vi "FTW-JSON-ObjectManip-AddPair-Boolean.vi"(0 "Input JSON Object":string, 5 "Key":string, 7 "Value":bool, 11 "error in":errorcluster) -> (4 "Output JSON Object":string, 15 "error out":errorcluster)   [LabVIEW 2013]
uses:
  FTW-JSON.lvclass
panel:
  # "Inputs"
  # "Outputs"
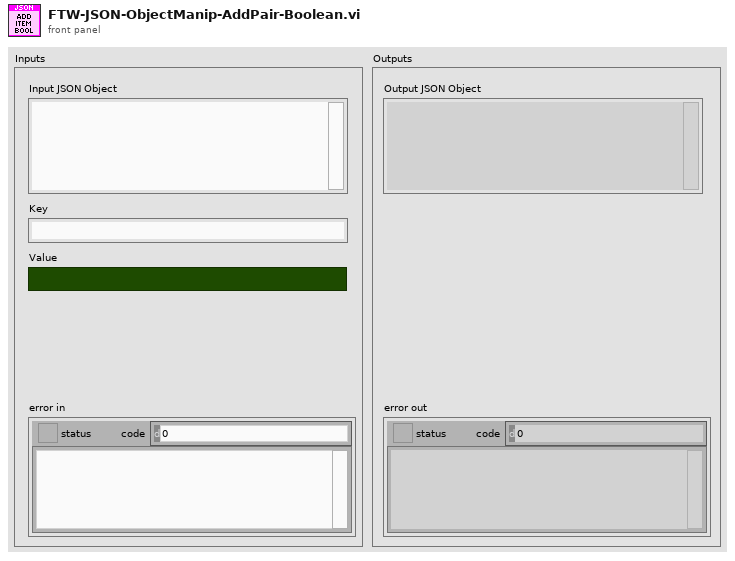
[diagram p1: front panel]
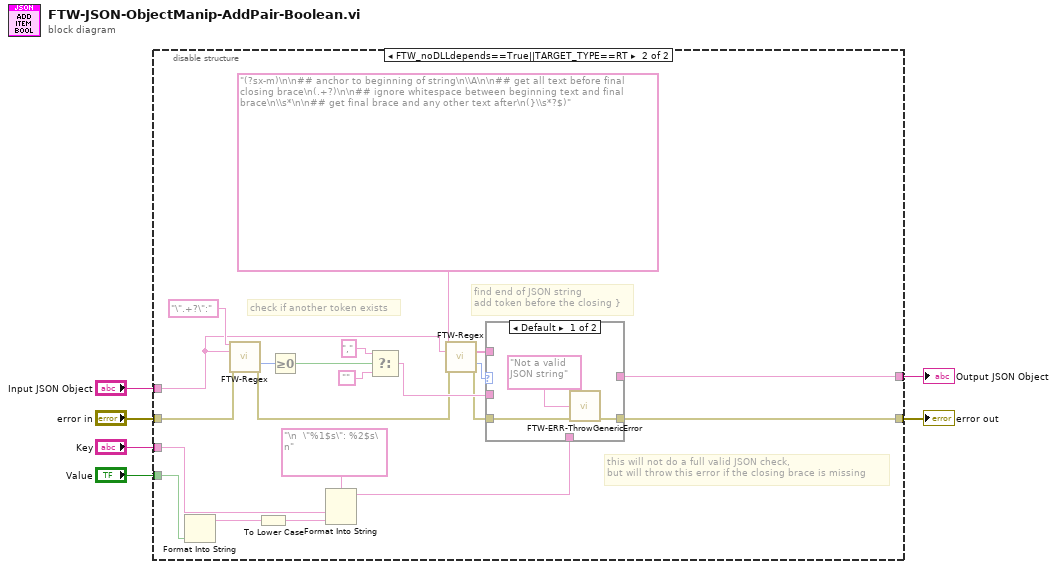
[diagram p0: block diagram]
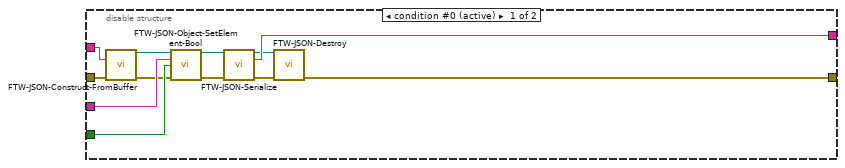
[diagram p2: hidden frame]
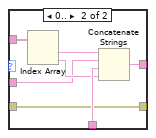
[diagram p3: hidden frame]
diagram:
  n1 = disable-structure shown="FTW_noDLLdepends==True||TARGET_TYPE==RT" {
    disable-tunnel: "Key" -> [w18 w31]
    disable-tunnel: "Value" -> [w17 w21]
    disable-tunnel: "Input JSON Object" -> [w16 w23]
    disable-tunnel: "error in" -> [w15 w30]
    disable-tunnel: [w14 w32] -> w2
    disable-tunnel: [w13 w33] -> w1
    frame condition #0 (active) {
      n2 = call "FTW-JSON-Construct-FromBuffer.vi"("JSON String (UTF-8)"=w16, "error in"=w15) -> ("JSON Object"=w10:refnum<class "FTW-JSON.lvclass">, "error out"=w8:errorcluster)  [unwired: 12 in]
      n3 = call "FTW-JSON-Object-SetElement-Bool.vi"("JSON Object"=w10, "Key"=w18, "Value"=w17, "error in"=w8) -> ("JSON Object out"=w9:refnum<class "FTW-JSON.lvclass">, "error out"=w7:errorcluster)  [unwired: 10 in]
      n4 = call "FTW-JSON-Serialize.vi"("JSON Object"=w9, "error in"=w7) -> ("JSON Object out"=w12:refnum<class "FTW-JSON.lvclass">, "JSON String (UTF-8)"=w13:string, "error out"=w11:errorcluster)  [unwired: 11 in]
      n5 = call "FTW-JSON-Destroy.vi"("JSON Object"=w12, "error in"=w11) -> ("error out"=w14:errorcluster)  [unwired: 13 in]
    }
    frame condition #1 {
      # "this will not do a full valid JSON check,\nbut will throw this error if the closing brace is missing"
      # "find end of JSON string\nadd token before the closing }"
      # "check if another token exists"
      n6 = Format Into String(w21) -> (resulting string=w20:string)  [unwired: 3 in, 1 out]
      n7 = call "FTW-Regex.vi"("Regular Expression"="\".+?\":" ("format string"), "Input String"=w23, "error in"=w30) -> ("Offset after Match"=w22:i32, "error out"=w28:errorcluster)  [unwired: 8 in, 3 out]
      n8 = To Lower Case(string=w20) -> (all lower case string=w19:string)
      n9 = Greater Or Equal To 0?(x=w22) -> (x >= 0?=w35:bool)
      n10 = Format Into String(format string="\n  \"%1$s\": %2$s\n", w31, w19) -> (resulting string=w38:string)  [unwired: 2 in, 1 out]
      n11 = Select(t="," ("format string"), s=w35, f="") -> (s? t:f=w39:string)
      n12 = call "FTW-Regex.vi"("Regular Expression"="(?sx-m)\n\n## anchor to beginning of string\n\\A\n\n## get all text before final closing brace\n(.+?)\n\n## ignore whitespace between beginning text and final brace\n\\s*\n\n## get final brace and any other text after\n(}\\s*?$)" ("format string"), "Input String"=w23, "error in"=w28) -> ("Submatches"=w25:string[], "Offset after Match"=w24:i32, "error out"=w27:errorcluster)  [unwired: 8 in, 2 out]
      n13 = case shown="Default" w24 {
        tunnel: w25 -> [_ w49]
        tunnel: w38 -> [_ w47]
        tunnel: [_ w45] -> w33
        tunnel: w27 -> [w42 w44]
        tunnel: w39 -> [_ w43]
        tunnel: [w41 w44] -> w32
        frame Default {
          n14 = call "FTW-ERR-ThrowGenericError.vi"("Error Message"="Not a valid JSON string", "error in"=w42) -> ("error out"=w41:errorcluster)  [unwired: 13 in]
        }
        frame 0.. {
          n15 = Index Array(array=w49) -> (element #1=w48:string, element #2=w46:string)  [unwired: 2 in]
          n16 = Concatenate Strings(w48, w43, w47, w46) -> (w45:string)
        }
      }
    }
  }
  "error out" <- w2
  "Output JSON Object" <- w1
